vi "Configuration--dialog .vi"(11 "Lv Proj Document Type:TAF Proj Config in":refnum<class "TAF Proj Config.lvclass">) -> (3 "Lv Proj Document Type:TAF Proj Config out":refnum<class "TAF Proj Config.lvclass">)   [LabVIEW 2021, in "TAF Proj Document Type.lvlib" / "TAF Proj Config.lvclass"]
uses:
  <vilib>/Wovalab/AntiDoc/Document Type/Add-ons/LabVIEW TAF Project/TAF Proj Config/TAF Proj Config.lvclass
  <vilib>/Utility/miscctls.llb/LVPointTypeDef.ctl
  <vilib>/Wovalab/AntiDoc/Document Type/Add-ons/LabVIEW TAF Project/TAF Proj Config/TAF Proj Config.lvclass/TAF Proj Config.ctl
  <vilib>/Wovalab/AntiDoc/Document Type/Add-ons/LabVIEW TAF Project/TAF Proj Config/Read Description Strip Tokens (string).vi
  <vilib>/Wovalab/AntiDoc/Document Type/Add-ons/LabVIEW TAF Project/TAF Proj Config/Read Lib Tokens (string).vi
  <vilib>/Wovalab/AntiDoc/Document Type/Add-ons/LabVIEW TAF Project/TAF Proj Config/Read List Dqmh Default Events.vi
  <vilib>/Wovalab/AntiDoc/Document Type/Add-ons/LabVIEW TAF Project/TAF Proj Config/Read Scan Dependencies.vi
  <vilib>/Wovalab/AntiDoc/Document Type/Add-ons/LabVIEW TAF Project/TAF Proj Config/Write Description Strip Tokens (string).vi
  <vilib>/Wovalab/AntiDoc/Document Type/Add-ons/LabVIEW TAF Project/TAF Proj Config/Write Lib Tokens (string).vi
  <vilib>/Wovalab/AntiDoc/Document Type/Add-ons/LabVIEW TAF Project/TAF Proj Config/Write List Dqmh Default Events.vi
  <vilib>/Wovalab/AntiDoc/Document Type/Add-ons/LabVIEW TAF Project/TAF Proj Config/Write Scan Dependencies.vi
  <vilib>/Wovalab/AntiDoc/Document Type/Add-ons/LabVIEW TAF Project/TAF Proj Config/Arrange Tokens String.vi
  <vilib>/Wovalab/AntiDoc/Utilities/Remove Empty Strings.vi
  <vilib>/AdvancedString/Join Strings.vi
  <vilib>/AdvancedString/Split String.vi
panel:
  in  "Description Strip Token":string caption="Description strip tokens"
  in  "Lib to Skip":string caption="Libraries to skip tokens"
  in  "List Default Dqmh Events":bool caption="List default DQMH events"
  in  "Scan Dependencies":bool caption="Scan for lib in Dependencies (this will increase generation process time)"
  in  "Cancel":bool
  in  "Apply":bool
  # "Notes:  -Tokens support regular expressions\n              - Tokens are case sensitive\n              - Add one token per line"
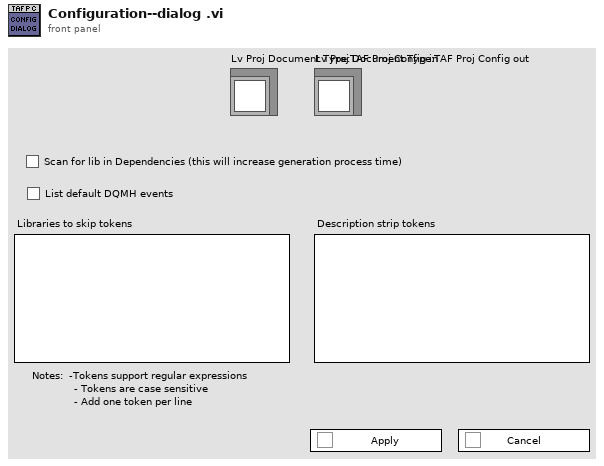
[diagram p1: front panel]
types:
  T1 = typedef "LVPointTypeDef.ctl" = cluster{"Horizontal":i16, "Vertical":i16}
  T2 = enum32{"Invalid", "Standard", "Closed", "Hidden", "Minimized", "Maximized"}
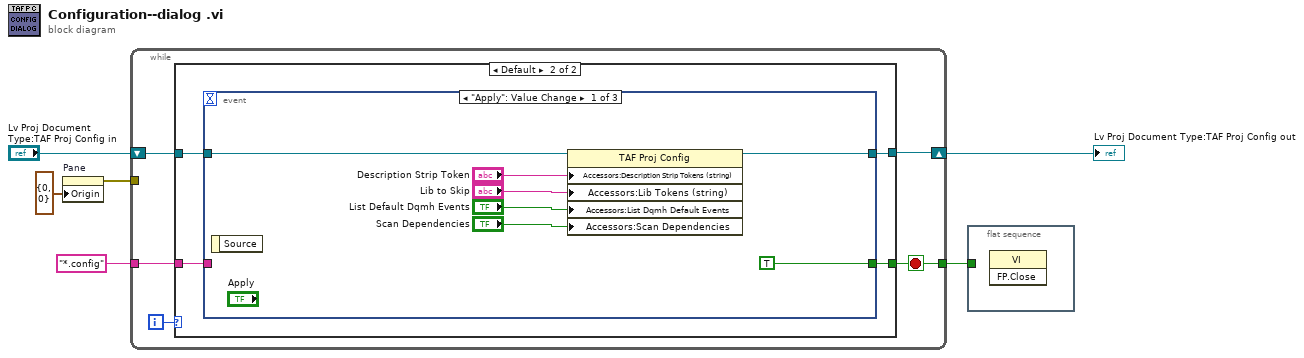
[diagram p0: block diagram]
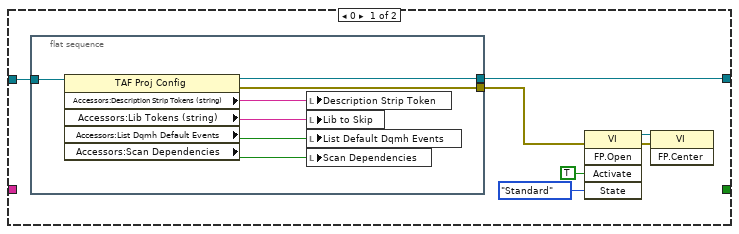
[diagram p2: hidden frame]
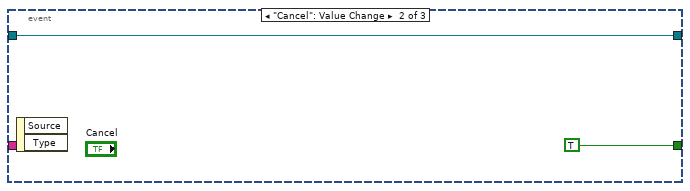
[diagram p3: hidden frame]
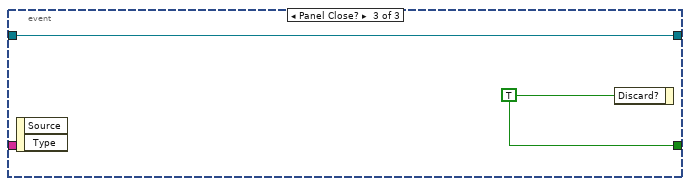
[diagram p4: hidden frame]
diagram:
  n1 = property on="Pane" class="Pane"("Origin"=T1 {"Horizontal"=0, "Vertical"=0}) -> (error out=w2:errorcluster)  [unwired: 2 in, 1 out]
  n2 = while {
    tunnel: [w11] -> w5
    shift-right: [w8] -> w3
    shift-left: "Lv Proj Document Type:TAF Proj Config in" -> [w9]
    tunnel: w2 -> [_]
    tunnel: "*.config" ("pattern (all files)") -> [w7]
    i -> [w10]
    stop <- w11 stop-if-true
    n3 = case shown="Default" w10 {
      tunnel: [_ w29] -> w11
      tunnel: w9 -> [w18 w28]
      tunnel: [w17 w27] -> w8
      tunnel: w7 -> [_ w26]
      frame 0 {
        n4 = flat-sequence {
          tunnel: w18 -> [w25]
          tunnel: [w20] -> w17
          tunnel: [w19] -> w12
          frame #0 {
            n5 = property class="TAF Proj Config"(reference=w25) -> (reference out=w20:refnum<class "TAF Proj Config.lvclass">, error out=w19:errorcluster, "Accessors:Description Strip Tokens (string)"=w21:string, "Accessors:Lib Tokens (string)"=w22:string, "Accessors:List Dqmh Default Events"=w23:bool, "Accessors:Scan Dependencies"=w24:bool)  [unwired: 1 in]
            n6 = local write "Description Strip Token"(w21) -> ()
            n7 = local write "Lib to Skip"(w22) -> ()
            n8 = local write "List Default Dqmh Events"(w23) -> ()
            n9 = local write "Scan Dependencies"(w24) -> ()
          }
        }
        n10 = invoke class="VI" method="FP.Open"(error in=w12, "Activate"=TRUE ("Activate?"), "State"=T2."Standard") -> (reference out=w14:refnum<vi>, error out=w13:errorcluster)  [unwired: 2 in, 3 out]
        n11 = invoke class="VI" method="FP.Center"(reference=w14, error in=w13) -> ()  [unwired: 1 in, 3 out]
      }
      frame Default {
        n12 = event shown="[0] \"Apply\": Value Change" {
          selector: _ -> [_ _ _]
          dyn-events: _ -> [_ _ _]
          timeout: _ -> [_ _ _]
          tunnel: [TRUE ("Discard?") TRUE w40] -> w29
          tunnel: w28 -> [w31 w37 w39]
          tunnel: [w30 w37 w39] -> w27
          tunnel: w26 -> [_ _ _]
          event "Apply": Value Change {
            n13 = event-data() -> ()  [unwired: 1 in, 1 out]
            n14 = property class="TAF Proj Config"(reference=w31, "Accessors:Description Strip Tokens (string)"="Description Strip Token", "Accessors:Lib Tokens (string)"="Lib to Skip", "Accessors:List Dqmh Default Events"="List Default Dqmh Events", "Accessors:Scan Dependencies"="Scan Dependencies") -> (reference out=w30:refnum<class "TAF Proj Config.lvclass">)  [unwired: 1 in, 1 out]
          }
          event "Cancel": Value Change {
            n15 = event-data() -> ()  [unwired: 1 in, 2 out]
          }
          event Panel Close? {
            w40 = TRUE ("Discard?")
            n16 = event-data() -> ()  [unwired: 1 in, 2 out]
            n17 = event-data("Discard?"=w40) -> ()  [unwired: 1 in, 1 out]
          }
        }
      }
    }
  }
  "Lv Proj Document Type:TAF Proj Config out" <- w3
  n18 = flat-sequence {
    tunnel: w5 -> [_]
    frame #0 {
      n19 = invoke class="VI" method="FP.Close"() -> ()  [unwired: 3 in, 3 out]
    }
  }
